vi "ELL9 Test Panel.vi"() -> ()   [LabVIEW 2020]
uses:
  <vilib>/Instr/_visa.llb/VISA Configure Serial Port (Instr).vi
panel:
  in  "Home Button":bool
  out "Number of positions":u8
  out "FW ID":string
  in  "COM Port":string[](array[string])
  in  "Quit":bool
  in  "Move position (Integer)":u8
  in  "Command":string
  out "Reply":string
  out "Command History":string
  out "Waiting for Reply":bool
  out "Current position":u8
  out "Last Error":errorcluster
  # "Example Commands:\n\nGet info for device\n0in\n\nGet device status\n0gs\n\nGo to home position (position 0)\n0ho0\n\nGo to position 0\n0ma00000000\n\nGo to position 1\n0ma00000020\n\nGo to position 2\n0ma00000040\n\nGo to position 3\n0ma00000060"
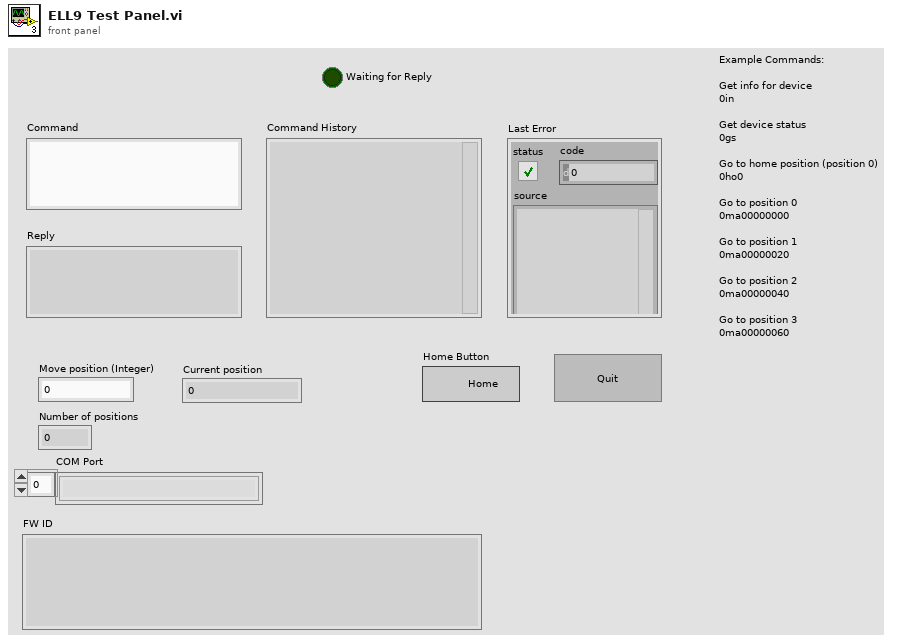
[diagram p1: front panel]
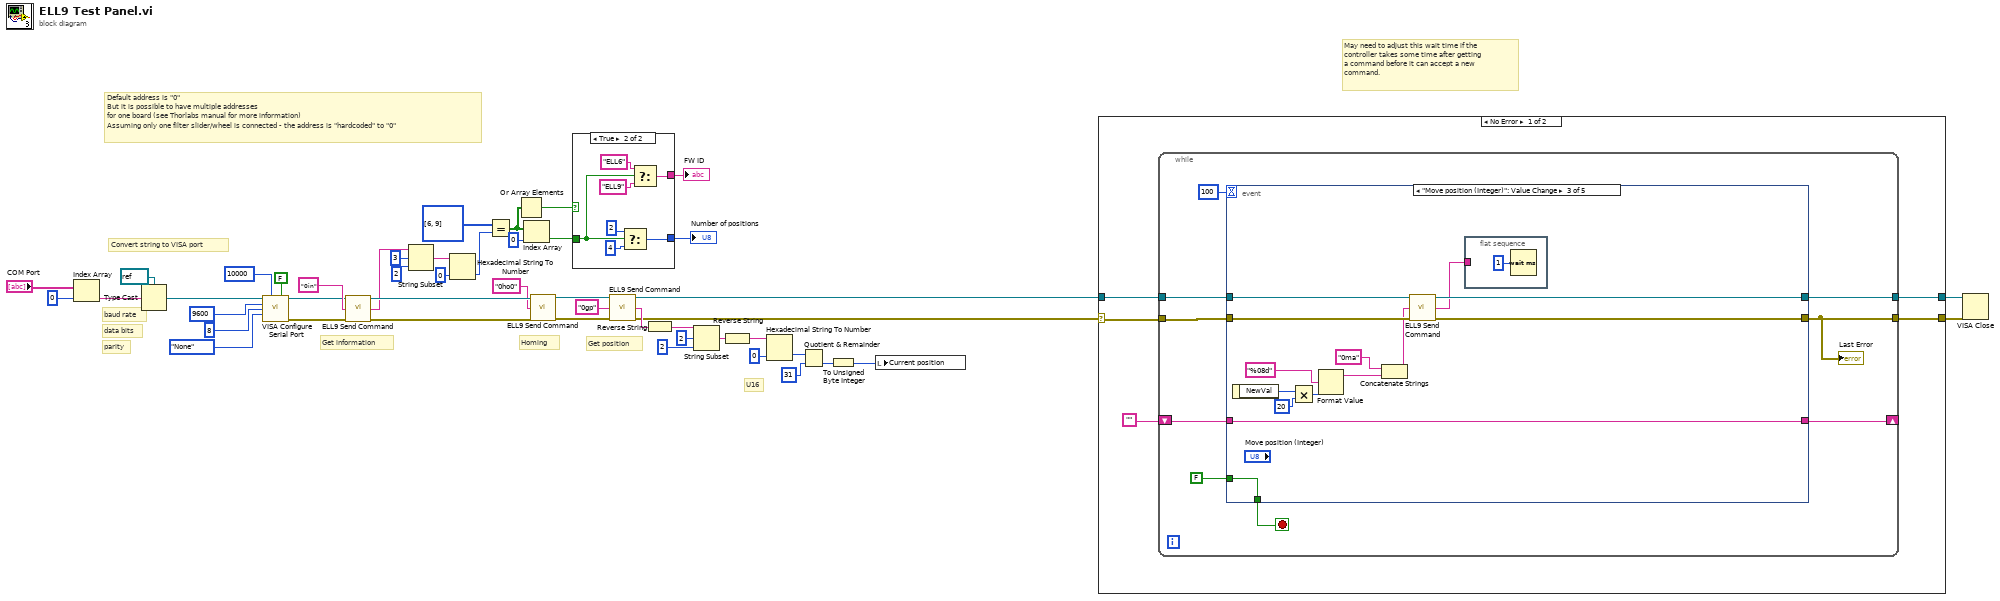
[diagram p0: block diagram]
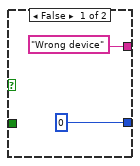
[diagram p2: hidden frame]
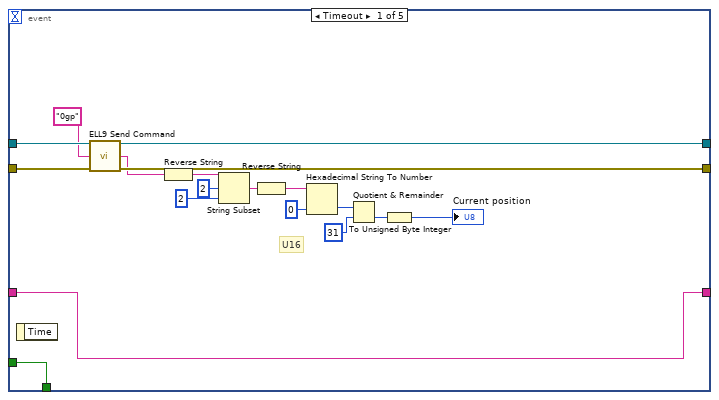
[diagram p3: hidden frame]
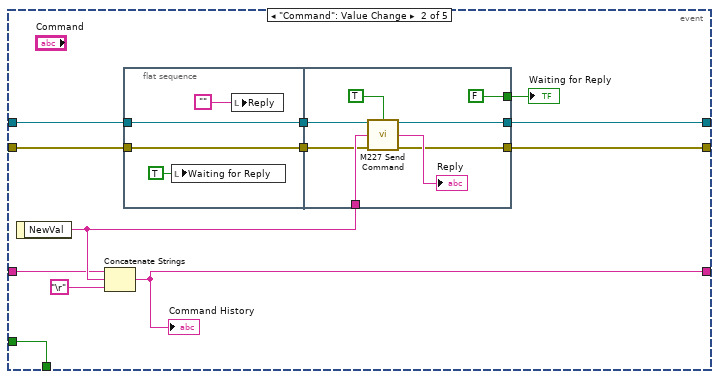
[diagram p4: hidden frame]
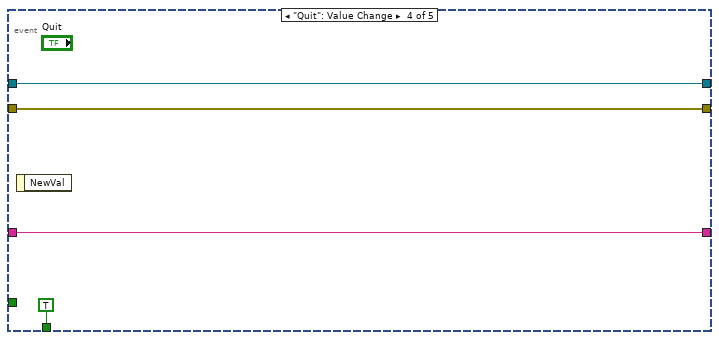
[diagram p5: hidden frame]
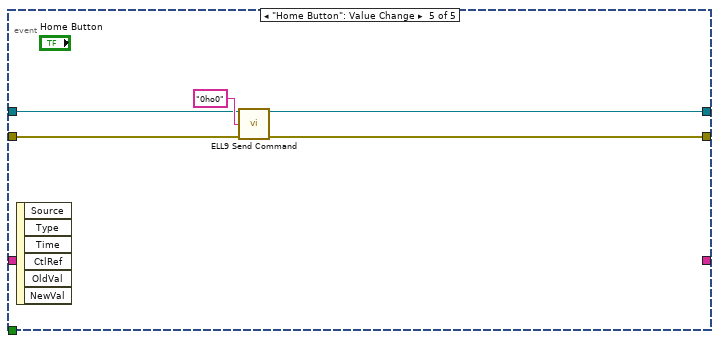
[diagram p6: hidden frame]
diagram:
  # "U16"
  # "Get position"
  # "Default address is \"0\"\nBut it is possible to have multiple addresses \nfor one board (see Thorlabs manual for more information)\nAssuming only one filter slider/wheel is connected - the address is \"hardcoded\" to \"0\""
  # "Get information"
  # "Homing"
  # "Convert string to VISA port"
  # "parity"
  # "data bits"
  # "baud rate"
  # "May need to adjust this wait time if the\ncontroller takes some time after getting\na command before it can accept a new\ncommand."
  n1 = Index Array(array="COM Port", index=0) -> (element=w38:string)
  n2 = Type Cast(type=refnum<visa-resource-name> refnum ("VISA resource name"), x=w38) -> (*(type *) &x=w36:refnum<visa-resource-name>)
  n3 = call-poly "VISA Configure Serial Port"("VISA resource name"=w36, "timeout (10sec)"=u32 10000, "Enable Termination\nChar (T)"=FALSE ("Enable Termination\nChar (T)"), "baud rate (9600)"=u32 9600 ("nbaud"), "data bits (8)"=u16 8, "parity (0:none)"=enum16{"None", "Odd", "Even", "Mark", "Space"}."None") -> ("VISA resource name out"=w28:refnum<visa-resource-name>, "error out"=w5:errorcluster)  [unwired: 4 in, 4 out]
  n4 = call "ELL9 Send Command.vi"("VISA Ref"=w28, "Command"="0in" ("write buffer"), "Error In"=w5) -> ("VISA Ref Dup"=w33:refnum<visa-resource-name>, "Reply"=w8:string, "Error Out"=w34:errorcluster)  [unwired: 9 in, 1 out]
  n5 = String Subset(string=w8, offset (0)=3, length (rest)=2 ("length (rest)")) -> (substring=w14:string)
  n6 = Hexadecimal String To Number(string=w14, default (0uL)=u16 0 ("default (0 U32)")) -> (number=w7:u16)  [unwired: 1 in, 1 out]
  n7 = Equal?(x=u16[] [6, 9] ("default (0 U32)"), y=w7) -> (x = y?=w12:bool[])
  n8 = Or Array Elements(Boolean array=w12) -> (logical OR=w13:bool)
  n9 = Index Array(array=w12, index=0) -> (element=w10:bool)
  n10 = call "ELL9 Send Command.vi"("VISA Ref"=w33, "Command"="0ho0" ("write buffer"), "Error In"=w34) -> ("VISA Ref Dup"=w30:refnum<visa-resource-name>, "Error Out"=w31:errorcluster)  [unwired: 9 in, 2 out]
  n11 = case shown="True" w13 {
    tunnel: w10 -> [_ w53]
    tunnel: ["Wrong device" ("write buffer") w54] -> w9
    tunnel: [u8 0 ("default (0 U32)") w50] -> w3
    frame False {
    }
    frame True {
      n12 = Select(t=u8 2 ("default (0 U32)"), s=w53, f=u8 4 ("default (0 U32)")) -> (s? t:f=w50:u8)
      n13 = Select(t="ELL6" ("write buffer"), s=w53, f="ELL9" ("write buffer")) -> (s? t:f=w54:string)
    }
  }
  "FW ID" <- w9
  "Number of positions" <- w3
  n14 = call "ELL9 Send Command.vi"("VISA Ref"=w30, "Command"="0gp" ("write buffer"), "Error In"=w31) -> ("VISA Ref Dup"=w4:refnum<visa-resource-name>, "Reply"=w25:string, "Error Out"=w1:errorcluster)  [unwired: 9 in, 1 out]
  n15 = Reverse String(1:w25) -> (0:w24:string)
  n16 = String Subset(string=w24, offset (0)=2, length (rest)=2 ("length (rest)")) -> (substring=w23:string)
  n17 = Reverse String(1:w23) -> (0:w20:string)
  n18 = Hexadecimal String To Number(string=w20, default (0uL)=u16 0 ("default (0 U32)")) -> (number=w22:u16)  [unwired: 1 in, 1 out]
  n19 = Quotient & Remainder(x=w22, y=u16 31) -> (floor(x/y)=w18:u16)  [unwired: 1 out]
  n20 = To Unsigned Byte Integer(number=w18) -> (unsigned 8bit integer=w2:u8)
  n21 = local write "Current position"(w2) -> ()
  n22 = case shown="No Error" w1 {
    selector: w1 -> [w60 w137]
    tunnel: w4 -> [w61 w138]
    tunnel: [w59 w138] -> w47
    tunnel: [w58 w137] -> w46
    frame No Error {
      n23 = while {
        tunnel: w61 -> [w68]
        tunnel: w60 -> [w67]
        tunnel: [w66] -> w59
        tunnel: [w63] -> w58
        shift-right: [w64] -> _
        shift-left: "" -> [w65]
        stop <- w69 stop-if-true
        n24 = event shown="[2] \"Move position (Integer)\": Value Change" {
          selector: _ -> [_ _ _ _ _]
          dyn-events: _ -> [_ _ _ _ _]
          timeout: 100 -> [_ _ _ _ _]
          tunnel: FALSE -> [w88 w100 w126 _ _]
          tunnel: [w88 w100 w126 TRUE _] -> w69
          tunnel: w68 -> [w87 w99 w125 w131 w134]
          tunnel: w67 -> [w86 w98 w124 w130 w135]
          tunnel: [w85 w94 w122 w131 w133] -> w66
          tunnel: [w84 w95 w121 w130 w132] -> w63
          tunnel: w65 -> [w83 w91 w120 w128 _]
          tunnel: [w83 w90 w120 w128 _] -> w64
          event Timeout {
            # "U16"
            n25 = event-data() -> ()  [unwired: 1 in, 1 out]
            n26 = call "ELL9 Send Command.vi"("VISA Ref"=w87, "Command"="0gp", "Error In"=w86) -> ("VISA Ref Dup"=w85:refnum<visa-resource-name>, "Reply"=w72:string, "Error Out"=w84:errorcluster)  [unwired: 9 in, 1 out]
            n27 = Reverse String(1:w72) -> (0:w79:string)
            n28 = String Subset(string=w79, offset (0)=2, length (rest)=2 ("length (rest)")) -> (substring=w78:string)
            n29 = Reverse String(1:w78) -> (0:w75:string)
            n30 = Hexadecimal String To Number(string=w75, default (0uL)=u16 0 ("default (0 U32)")) -> (number=w77:u16)  [unwired: 1 in, 1 out]
            n31 = Quotient & Remainder(x=w77, y=u16 31) -> (floor(x/y)=w73:u16)  [unwired: 1 out]
            n32 = To Unsigned Byte Integer(number=w73) -> (unsigned 8bit integer=→"Current position":u8)
          }
          event "Command": Value Change {
            n33 = event-data() -> ("NewVal"=w93:string)  [unwired: 1 in]
            n34 = Concatenate Strings(w91, w93, "\r") -> (w90:string)
            "Command History" <- w90
            n35 = flat-sequence {
              tunnel: w98 -> [w103]
              tunnel: w99 -> [w104]
              tunnel: [w104] -> w97
              tunnel: [w103] -> w96
              tunnel: w93 -> [w110]
              tunnel: w97 -> [w112]
              tunnel: w96 -> [w109]
              tunnel: [w107] -> w95
              tunnel: [w106] -> w94
              tunnel: [FALSE] -> w89
              frame #0 {
                n36 = local write "Waiting for Reply"(TRUE ("Waiting for Cmd")) -> ()
                n37 = local write "Reply"("") -> ()
              }
              frame #1 {
                n38 = call "M227 Send Command.vi"("VISA Ref"=w112, "Wait for Reply (T)"=TRUE, "Command"=w110, "Error In"=w109) -> ("VISA Ref Dup"=w106:refnum<visa-resource-name>, "Reply"=→"Reply":string, "Error Out"=w107:errorcluster)  [unwired: 9 in]
              }
            }
            "Waiting for Reply" <- w89
          }
          event "Move position (Integer)": Value Change {
            n39 = event-data() -> ("NewVal"=w119:u8)  [unwired: 1 in]
            n40 = Multiply(x=w119, y=u8 20) -> (x*y=w117:u8)
            n41 = Format Value(format string="%08d", value (0)=w117) -> (output string=w115:string)  [unwired: 1 in]
            n42 = Concatenate Strings("0ma" ("string"), w115) -> (w113:string)
            n43 = call "ELL9 Send Command.vi"("VISA Ref"=w125, "Command"=w113, "Error In"=w124) -> ("VISA Ref Dup"=w122:refnum<visa-resource-name>, "Reply"=w116:string, "Error Out"=w121:errorcluster)  [unwired: 9 in, 1 out]
            n44 = flat-sequence {
              tunnel: w116 -> [_]
              frame #0 {
                n45 = Wait (ms)(milliseconds to wait=u32 1) -> ()  [unwired: 1 out]
              }
            }
          }
          event "Quit": Value Change {
            n46 = event-data() -> ()  [unwired: 1 in, 1 out]
          }
          event "Home Button": Value Change {
            n47 = event-data() -> ()  [unwired: 1 in, 6 out]
            n48 = call "ELL9 Send Command.vi"("VISA Ref"=w134, "Command"="0ho0" ("write buffer"), "Error In"=w135) -> ("VISA Ref Dup"=w133:refnum<visa-resource-name>, "Error Out"=w132:errorcluster)  [unwired: 9 in, 2 out]
          }
        }
        "Last Error" <- w63
      }
    }
    frame Error {
    }
  }
  n49 = VISA Close(VISA resource name=w47, error in (no error)=w46) -> ()  [unwired: 1 out]
